vi "lvEtherbone.device_open.vi"(0 "eb_socket_ID":i32, 1 "ip_port":string, 2 "proposed_port_widths":T2=15 items=["EB_DATA8"=1, "EB_DATA16"=2, "EB_DATA32"=4, "EB_DATA64"=8, "EB_DATAX"=15], 3 "timeout [ms]":i32=1000, 4 "proposed_address_widths":T1=15 items=["EB_ADDR8"=1, "EB_ADDR16"=2, "EB_ADDR32"=4, "EB_ADDR64"=8, "EB_ADDRX"=15], 5 "error in (no error)":errorcluster) -> (13 "eb_status":T3, 14 "eb_socket_ID out":i32, 15 "eb_device_ID":i32, 17 "timed out?":bool, 19 "error out":errorcluster)   [LabVIEW 2009, in "lvEtherbone.lvlib"]
doc: "//-----------------------------------------------------------------------------------\n// author : Dietrich Beck, GSI-Darmstadt\n// purpose : Open a remote Etherbone device.\n// This resolves the address and performs Etherbone end-point discovery.\n// From the mask of proposed bus address widths, one will be selected.\n// From the mask of proposed bus port widths, one will be selected.\n// The timeout value has a granularity of 3000 milliseconds.\n// The default port is taken as 0xEBD0.\n// returns : lveb_status_t\n//-----------------------------------------------------------------------------------\nETHERBONE_API int lveb_device_open( int eb_socketID, //Etherbone socket ID\n char *ip_port, //IP port in the format \"IP:PORT\"\n int proposed_addr_widths, //widths of addresses (range)\n int proposed_port_widths, //widths of ports (\"data type\")\n int timeout, //timeout [ms]\n int *eb_deviceID //Etherbone device ID\n );"
uses:
  lvEtherbone.lvlib
  lvEtherbone.lveb_status_t.ctl
  lvEtherbone.eb_portWidth_t.ctl
  lvEtherbone.eb_addressWidth_t.ctl
  bin/lvEtherbone.dll
panel:
  in  "eb_status_t":T3
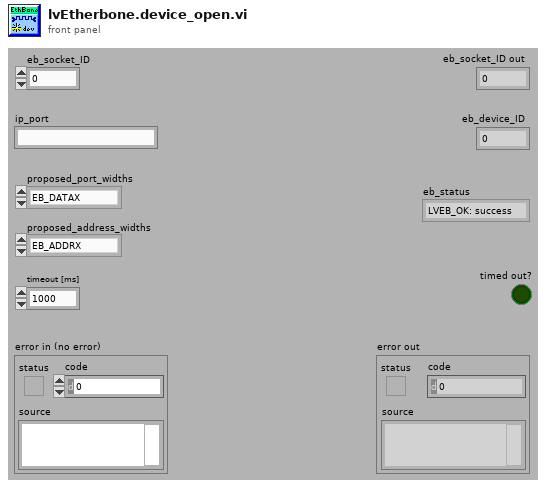
[diagram p1: front panel]
types:
  T1 = typedef "lvEtherbone.lvlib/lvEtherbone.eb_addressWidth_t.ctl" = u32
  T2 = typedef "lvEtherbone.lvlib/lvEtherbone.eb_portWidth_t.ctl" = u32
  T3 = typedef "lvEtherbone.lvlib/lvEtherbone.lveb_status_t.ctl" = enum32{"LVEB_OK: success", "LVEB_UNKNOWN: unknown error", "LVEB_OS: operating system forbids access", "LVEB_PORT: port in use or unavailable", "LVEB_ID: ID invalid or out of resources", "LVEB_SOCKET: socket invalid or unavailable", "LVEB_EB: remote address is not Etherbone conformant", "LVEB_IP: bad format or network address", "LVEB_PORTWIDTH: port width error", "LVEB_DEVICEBUSY: Etherbone device still busy", "LVEB_DEVICEFAIL: operation on Wishbone device failed", "LVEB_DEVICEEXIST: Etherbone device already exists, overlaps, or does not exist", "LVEB_TIMEDOUT: a timeout occurred", "LVEB_OVERFLOW: payload of Etherbone exceeded", "LVEB_ADDRESS: bad address", "LVEB_ADDRESSWIDTH: address width error"}
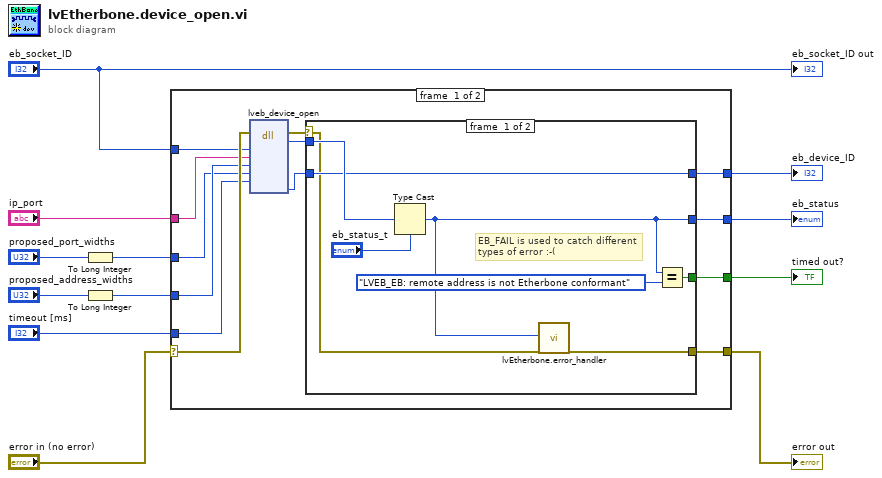
[diagram p0: block diagram]
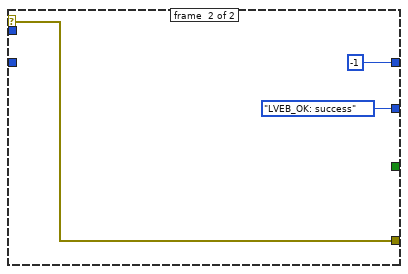
[diagram p2: hidden frame]
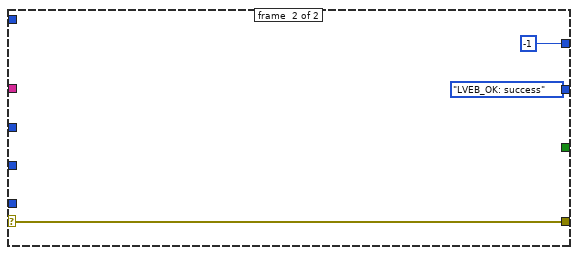
[diagram p3: hidden frame]
diagram:
  n1 = To Long Integer(number="proposed_port_widths") -> (32bit integer=w5:i32)
  n2 = To Long Integer(number="proposed_address_widths") -> (32bit integer=w3:i32)
  n3 = case shown="No Error" "error in (no error)" {
    selector: "error in (no error)" -> [w25 w39]
    tunnel: [w22 w39] -> w11
    tunnel: "eb_socket_ID" -> [w17 _]
    tunnel: "ip_port" -> [w19 _]
    tunnel: [w23 lvEtherbone.lveb_status_t."LVEB_OK: success" ("eb_status_t")] -> w9
    tunnel: [w21 -1 ("eb_socket_ID")] -> w8
    tunnel: w5 -> [w13 _]
    tunnel: w3 -> [w14 _]
    tunnel: "timeout [ms]" -> [w16 _]
    tunnel: [w15 _] -> w1
    frame #0 {
      n4 = dll-call lib="F:/beck/Project/BEL/SCC/etherbone-core/api/lvEtherbone/bin/lvEtherbone.*" fn="lveb_device_open"(error in=w25, "eb_socket_ID"=w17, "ip_port"=w19, "proposed_addr_widths"=w14, "proposed_port_widths"=w13, "timeout"=w16) -> (error out=w20:errorcluster, "eb_status"=w24:i32, "eb_device_ID"=w18:i32)  [unwired: 8 in, 1 out]
      n5 = case shown="No Error" w20 {
        selector: w20 -> [w29 w36]
        tunnel: w24 -> [w33 _]
        tunnel: [w28 lvEtherbone.lveb_status_t."LVEB_OK: success" ("eb_status_t")] -> w23
        tunnel: [w30 w36] -> w22
        tunnel: w18 -> [w32 _]
        tunnel: [w32 -1 ("eb_socket_ID")] -> w21
        tunnel: [w26 _] -> w15
        frame #0 {
          # "EB_FAIL is used to catch different\ntypes of error :-("
          n6 = Type Cast(type="eb_status_t", x=w33) -> (*(type *) &x=w28:T3)
          n7 = call "lvEtherbone.error_handler.vi"("eb_status"=w28, "error in"=w29) -> ("error out"=w30:errorcluster)  [unwired: 17 in]
          n8 = Equal?(x=w28, y=lvEtherbone.lveb_status_t."LVEB_EB: remote address is not Etherbone conformant") -> (x = y?=w26:bool)
        }
        frame #1 {
        }
      }
    }
    frame #1 {
    }
  }
  "error out" <- w11
  "eb_status" <- w9
  "eb_device_ID" <- w8
  "timed out?" <- w1
  "eb_socket_ID out" <- "eb_socket_ID"
